vi "4155C Config VSU2 Stress v3.0.vi"(0 "VISA session":refnum<visa-resource-name>, 1 "Display on/off":bool, 2 "VSU2":dbl min=0.0 max=100000000000.0 format="%.15e", 3 "error in (no error)":errorcluster, 4 "VSU2 Stress - Source/Common":u32(ring) items=["SMU1  ", "SMU2  ", "SMU3  ", "SMU4  ", "SMU5  ", "SMU6  ", "VSU1  "]) -> (5 "dup VISA resource name":refnum<visa-resource-name>, 6 "error out":errorcluster)   [LabVIEW 2016]
panel:
  # "This program uses VSU2 to stress the device. Hence the only freedom allowed is on choosing which SMU to use for ground."
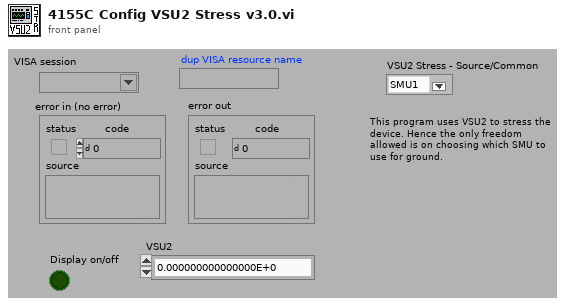
[diagram p1: front panel]
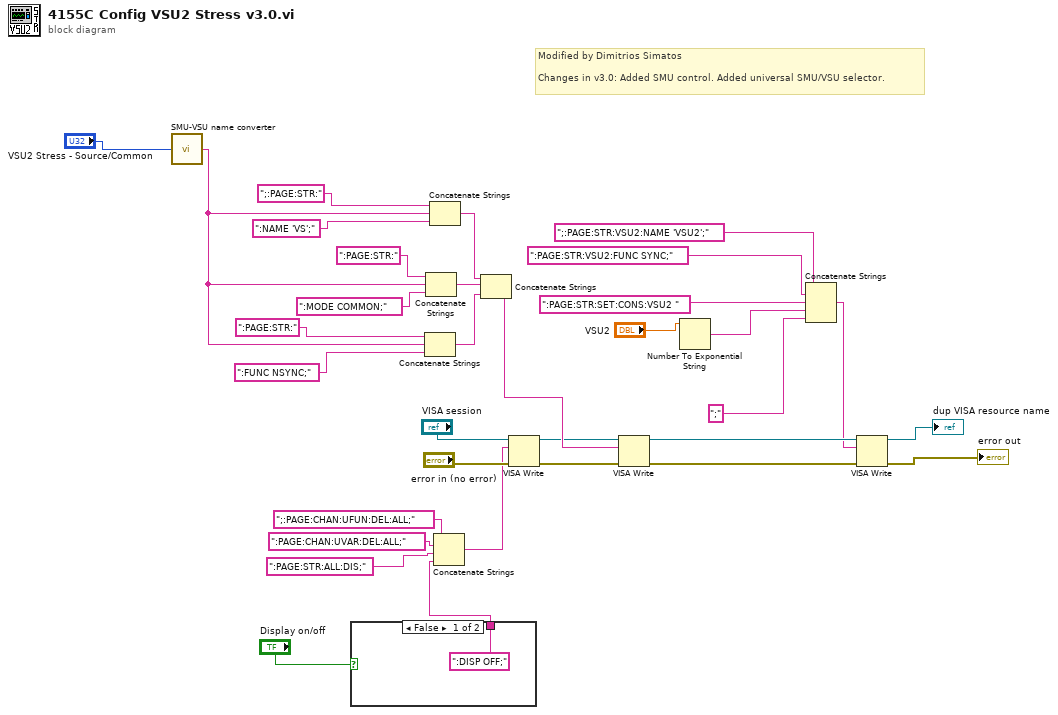
[diagram p0: block diagram]
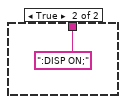
[diagram p2: hidden frame]
diagram:
  # "Modified by Dimitrios Simatos\n\nChanges in v3.0: Added SMU control. Added universal SMU/VSU selector."
  n1 = call "SMU-VSU name converter.vi"("unit to configure"="VSU2 Stress - Source/Common") -> ("SMU/VSU to be configured"=w1:string)
  n2 = case shown="False" "Display on/off" {
    tunnel: [":DISP OFF;" ("write buffer (\"\")") ":DISP ON;" ("write buffer (\"\")")] -> w27
    frame False {
    }
    frame True {
    }
  }
  n3 = Concatenate Strings(":PAGE:STR:", w1, ":FUNC NSYNC;") -> (w4:string)
  n4 = Concatenate Strings(":PAGE:STR:", w1, ":MODE COMMON;") -> (w7:string)
  n5 = Concatenate Strings(";:PAGE:STR:", w1, ":NAME 'VS';") -> (w10:string)
  n6 = Concatenate Strings(";:PAGE:CHAN:UFUN:DEL:ALL;", ":PAGE:CHAN:UVAR:DEL:ALL;", ":PAGE:STR:ALL:DIS;", w27) -> (w28:string)
  n7 = Concatenate Strings(w10, w7, w4) -> (w19:string)
  n8 = VISA Write(VISA resource name="VISA session", write buffer=w28, error in (no error)="error in (no error)") -> (VISA resource name out=w18:refnum<visa-resource-name>, error out=w17:errorcluster)  [unwired: 1 out]
  n9 = VISA Write(VISA resource name=w18, write buffer=w19, error in (no error)=w17) -> (VISA resource name out=w33:refnum<visa-resource-name>, error out=w32:errorcluster)  [unwired: 1 out]
  n10 = Number To Exponential String(number="VSU2") -> (E-format string=w21:string)  [unwired: 3 in]
  n11 = Concatenate Strings(";:PAGE:STR:VSU2:NAME 'VSU2';", ":PAGE:STR:VSU2:FUNC SYNC;", ":PAGE:STR:SET:CONS:VSU2 ", w21, ";" ("Substring")) -> (w16:string)
  n12 = VISA Write(VISA resource name=w33, write buffer=w16, error in (no error)=w32) -> (VISA resource name out=→"dup VISA resource name":refnum<visa-resource-name>, error out=→"error out":errorcluster)  [unwired: 1 out]
